vi "analyze data.vi"() -> ()   [LabVIEW 2014]
uses:
  <vilib>/Analysis/baseanly.llb/Mean (DBL).vi
  <vilib>/gmath/SpecialFunctions.llb/Factorial.vi
  <vilib>/Utility/file.llb/Read From Spreadsheet File (DBL).vi
  <vilib>/imath/engines/lvmath2/RunTimeEngine/Managers/WorkSpace/UID Generator.vi
  <vilib>/imath/engines/lvmath2/RunTimeEngine/RunTimeType/NIMS_RunTimeType_From StrictType (excl LVString).vi
  <instcachedir>/0/NIMS_RunTimeType_From StrictType (excl LVString)_15A5391EEA9C4AACB9955AC755B83D29.lvgen/NIMS_RunTimeType_From StrictType (excl LVString)_15A5391EEA9C4AACB9955AC755B83D29_000.vi
  <vilib>/imath/engines/lvmath2/RunTimeEngine/LocalVariableDefStatement/MC_LocalVariableDefStatement_Display.vi
  <vilib>/imath/engines/lvmath2/RunTimeEngine/BuiltInFunctions/max/1 input/NIMS_max(RV).vi
  <instcachedir>/0/NIMS_max(RV)_237633DB1D604D5BA7001287DF3C7957.lvgen/NIMS_max(RV)_237633DB1D604D5BA7001287DF3C7957_000.vi
  <vilib>/imath/engines/lvmath2/RunTimeEngine/Managers/SymbolTable/Clear UID.vi
  <vilib>/imath/engines/lvmath2/RunTimeEngine/NodeEndStatement/NIMS_NodeEndStatement_Output.vi
  <instcachedir>/0/NIMS_NodeEndStatement_Output_53EC0D466D134D7ABD903AC30B43404B.lvgen/NIMS_NodeEndStatement_Output_53EC0D466D134D7ABD903AC30B43404B_005.vi
  <instcachedir>/0/NIMS_NodeEndStatement_Output_53EC0D466D134D7ABD903AC30B43404B.lvgen/NIMS_NodeEndStatement_Output_53EC0D466D134D7ABD903AC30B43404B_004.vi
  <vilib>/imath/engines/lvmath2/RunTimeEngine/ErrorHandling/NIMS_Finalize Error.vi
  <vilib>/Analysis/NI_AALBase.lvlib
  <vilib>/gmath/NI_Gmath.lvlib
  <vilib>/imath/engines/lvmath2/RunTimeEngine/Managers/SymbolTable/NIMS_WorkSpace.lvlib
panel:
  out "?":dbl=44.2093023255814
  out "XY Graph 2":cluster{"X Values":dbl[], "yout":dbl[]}[](graph)=[{"X Values"=[3.05, 9.15, 15.25, 21.35, 27.45, 33.55, 39.65, 45.75, 51.85, 57.95], "yout"=[1.0, 0.0, 0.0, 0.0, 6.0, 30.0, 83.0, 101.0, 64.0, 16.0]}, {"X Values"=[1.0, 2.0, 3.0, 4.0, 5.0, 6.0, 7.0, 8.0, 9.0, 10.0, 11.0, 12.0, 13.0, 14.0, 15.0, 16.0, 17.0, 18.0, 19.0, 20.0, 21.0, 22.0, 23.0, 24.0, 25.0, 26.0, 27.0, 28.0, 29.0, 30.0, 31.0, 32.0, 33.0, 34.0, 35.0, 36.0, 37.0, 38.0, 39.0, 40.0, 41.0, 42.0, 43.0, 44.0, 45.0, 46.0, 47.0, 48.0, 49.0, 50.0, 51.0, 52.0, 53.0, 54.0, 55.0, 56.0, 57.0, 58.0, 59.0, 60.0], "yout"=[4.697137632968925e-15, 1.0382858884039449e-13, 1.530063158027829e-12, 1.691075618262153e-11, 1.4952254652634198e-10, 1.101714577312311e-09, 6.958004689271438e-09, 3.845106661135175e-08, 1.8887720317359093e-07, 8.350129377511543e-07, 3.3559399464375147e-06, 1.2363646973212627e-05, 4.204524668350126e-05, 0.00013277078728461114, 0.00039131359167138887, 0.0010812313048943463, 0.002811793037762178, 0.00690596713796628, 0.016068841529099022, 0.035519613659089816, 0.07477606374964532, 0.1502635276829554, 0.2888280749497454, 0.5320369868987074, 0.9408393600878537, 1.599763527305018, 2.619423312150594, 4.135817040197906, 6.304882272186222, 9.29114821660931, 13.250167111608626, 18.30564511567442, 24.52363027829251, 31.88742897334752, 40.27774251052069, 49.462524878875854, 59.10010043667066, 68.75721599149993, 77.94124484188515, 86.14320142117656, 92.88611792493289, 97.77215402840388, 100.52183061546553, 101.0, 99.22532299741601, 95.36265875535283, 89.70035343588606, 82.61645924497063, 74.53910252714248, 65.90643437399899, 57.13093102825904, 48.57151157635083, 40.51533282432774, 33.169529586152905, 26.66185020857364, 21.04824636482496, 16.32505766606783, 12.443438100719709, 9.323995202786033, 6.87012204670397]}]
  in  "Constant Data":path=path "U:/LabView/week8/constant.txt"
  out "Mean Lifetime":dbl=140.7967398239417
  out "XY Graph":cluster{"all rows":dbl[], "Array":dbl[]}[](graph)=[{"all rows"=[0.0, 1.0, 2.0, 3.0, 4.0, 5.0, 6.0, 7.0, 8.0, 9.0, 10.0, 11.0, 12.0, 13.0, 14.0, 15.0, 16.0, 17.0, 18.0, 19.0, 20.0, 21.0, 22.0, 23.0, 24.0, 25.0, 26.0, 27.0, 28.0, 29.0, 30.0, 31.0, 32.0, 33.0, 34.0, 35.0, 36.0, 37.0, 38.0, 39.0, 40.0, 41.0, 42.0, 43.0, 44.0, 45.0, 46.0, 47.0, 48.0, 49.0, 50.0, 51.0, 52.0, 53.0, 54.0, 55.0, 56.0, 57.0, 58.0, 59.0, 60.0, 61.0, 62.0, 63.0, 64.0, 65.0, 66.0, 67.0, 68.0, 69.0, 70.0, 71.0, 72.0, 73.0, 74.0, 75.0, 76.0, 77.0, 78.0, 79.0, 80.0, 81.0, 82.0, 83.0, 84.0, 85.0, 86.0, 87.0, 88.0, 89.0, 90.0, 91.0, 92.0, 93.0, 94.0, 95.0, 96.0, 97.0, 98.0, 99.0, 100.0, 101.0, 102.0, 103.0, 104.0, 105.0, 106.0, 107.0, 108.0, 109.0, 110.0, 111.0, 112.0, 113.0, 114.0, 115.0, 116.0, 117.0, 118.0, 119.0, 120.0, 121.0, 122.0, 123.0, 124.0, 125.0, 126.0, 127.0, 128.0, 129.0, 130.0, 131.0, 132.0, 133.0, 134.0, 135.0, 136.0, 137.0, 138.0, 139.0, 140.0, 141.0, 142.0, 143.0, 144.0, 145.0, 146.0, 147.0, 148.0, 149.0, 150.0, 151.0, 152.0, 153.0, 154.0, 155.0, 156.0, 157.0, 158.0, 159.0, 160.0, 161.0, 162.0, 163.0, 164.0, 165.0, 166.0, 167.0, 168.0, 169.0, 170.0, 171.0, 172.0, 173.0, 174.0, 175.0, 176.0, 177.0, 178.0, 179.0, 180.0, 181.0, 182.0, 183.0, 184.0, 185.0, 186.0, 187.0, 188.0, 189.0, 190.0, 191.0, 192.0, 193.0, 194.0, 195.0, 196.0, 197.0, 198.0, 199.0, 200.0, 201.0, 202.0, 203.0, 204.0, 205.0, 206.0, 207.0, 208.0, 209.0, 210.0, 211.0, 212.0, 213.0, 214.0, 215.0, 216.0, 217.0, 218.0, 219.0, 220.0, 221.0, 222.0, 223.0, 224.0, 225.0, 226.0, 227.0, 228.0, 229.0, 230.0, 231.0, 232.0, 233.0, 234.0, 235.0, 236.0, 237.0, 238.0, 239.0, 240.0, 241.0, 242.0, 243.0, 244.0, 245.0, 246.0, 247.0, 248.0, 249.0, 250.0, 251.0, 252.0, 253.0, 254.0, 255.0, 256.0, 257.0, 258.0, 259.0, 260.0, 261.0, 262.0, 263.0, 264.0, 265.0, 266.0, 267.0, 268.0, 269.0, 270.0, 271.0, 272.0, 273.0, 274.0, 275.0, 276.0, 277.0, 278.0, 279.0, 280.0, 281.0, 282.0, 283.0, 284.0, 285.0, 286.0, 287.0, 288.0, 289.0, 290.0, 291.0, 292.0, 293.0, 294.0, 295.0, 296.0, 297.0, 298.0, 299.0, 300.0], "Array"=[33.48144002446238, 33.24448268334883, 33.00920235437892, 32.775587168877394, 32.54362534216689, 32.313305172973415, 32.08461504283611, 31.857543415521167, 31.63207883643986, 31.408209932070736, 31.185925409385867, 30.96521405528119, 30.746064736010855, 30.528466396625596, 30.31240806041504, 30.097878828354023, 29.884867878552765, 29.673364465710968, 29.463357920575785, 29.25483764940359, 29.04779313342559, 28.842213928317204, 28.638089663671213, 28.435410042474604, 28.23416484058916, 28.034343906235687, 27.835937159481933, 27.638934591734085, 27.44332626523189, 27.249102312547365, 27.05625293608701, 26.86476840759759, 26.674639067675397, 26.48585532527895, 26.29840765724523, 26.112286607809242, 25.927482788127033, 25.74398687580208, 25.56178961441502, 25.380881813056703, 25.201254345864577, 25.02289815156232, 24.84580423300275, 24.669963656713954, 24.49536755244867, 24.3220071127368, 24.149873592441132, 23.97895830831619, 23.809252638570207, 23.640748022430206, 23.473435959710155, 23.30730801038216, 23.142355794150735, 22.97857099003003, 22.815945335924102, 22.654470628210138, 22.494138721324603, 22.334941527352356, 22.176871015618655, 22.019919212284037, 21.864078199942103, 21.709340117220098, 21.555697158382372, 21.403141572936605, 21.25166566524284, 21.10126179412526, 20.951922372486774, 20.80363986692624, 20.65640679735847, 20.510215736636894, 20.365059310178896, 20.220930195593805, 20.077821122313505, 19.935724871225712, 19.79463427430976, 19.654542214275047, 19.515441624201983, 19.377325487185505, 19.24018683598112, 19.104018752653428, 18.96881436822717, 18.834566862340697, 18.701269462901937, 18.56891544574677, 18.437498134299844, 18.30701089923774, 18.177447158154596, 18.048800375230044, 17.921064060899507, 17.794231771526835, 17.668297109079266, 17.54325372080466, 17.419095298911067, 17.295815580248494, 17.17340834599299, 17.051867421332922, 16.931186675157495, 16.81136001974748, 16.69238141046808, 16.57424484546407, 16.456944365356982, 16.340474052944508, 16.224828032902007, 16.110000471486128, 15.995985576240512, 15.882777595703615, 15.770370819118556, 15.658759576145052, 15.547938236573373, 15.437901210040335, 15.328642945747278, 15.220157932180078, 15.112440696831099, 15.005485805923149, 14.899287864135378, 14.793841514331083, 14.689141437287507, 14.585182351427475, 14.481959012552998, 14.37946621358071, 14.277698784279199, 14.176651591008207, 14.076319536459653, 13.976697559400504, 13.87778063441747, 13.779563771663474, 13.682042016605976, 13.585210449777005, 13.489064186525031, 13.39359837676853, 13.298808204751346, 13.204688888799744, 13.111235681081212, 13.01844386736495, 12.92630876678406, 12.834825731599434, 12.743990146965272, 12.653797430696324, 12.564243033036707, 12.47532243643042, 12.387031155293437, 12.299364735787451, 12.212318755595184, 12.125888823697311, 12.04007058015096, 11.95485969586977, 11.870251872405513, 11.786242841731255, 11.702828366026065, 11.620004237461234, 11.537766277988005, 11.456110339126832, 11.375032301758079, 11.294528075914267, 11.214593600573732, 11.135224843455775, 11.056417800817258, 10.978168497250623, 10.900472985483372, 10.82332734617894, 10.74672768773897, 10.670670146107023, 10.595150884573652, 10.52016609358285, 10.445711990539879, 10.371784819620473, 10.298380851581358, 10.225496383572143, 10.153127738948518, 10.081271267086803, 10.009923343199779, 9.939080368153839, 9.86873876828744, 9.798894995230812, 9.729545525726982, 9.660686861454026, 9.592315528848614, 9.524428078930763, 9.45702108712988, 9.390091153111992, 9.32363490060823, 9.257648977244495, 9.192130054372369, 9.127074826901191, 9.06248001313133, 8.998342354588646, 8.934658615860117, 8.871425584430623, 8.8086400705209, 8.746298906926627, 8.68439894885865, 8.62293707378436, 8.56191018127016, 8.501315192825087, 8.441149051745484, 8.381408722960836, 8.322091192880658, 8.263193469242466, 8.204712580960841, 8.146645577977546, 8.088989531112729, 8.031741531917133, 7.974898692525403, 7.918458145510397, 7.862417043738543, 7.806772560226216, 7.7515218879971295, 7.696662239940735, 7.642190848671633, 7.588104966389972, 7.534401864742834, 7.481078834686598, 7.428133186350296, 7.375562248899908, 7.323363370403647, 7.271533917698167, 7.220071276255748, 7.1689728500523975, 7.1182360614369, 7.067858351000779, 7.017837177449201, 6.968170017472771, 6.91885436562025, 6.869887734172157, 6.821267653015293, 6.772991669518124, 6.725057348407065, 6.677462271643629, 6.630204038302449, 6.583280264450172, 6.536688583025188, 6.49042664371824, 6.444492112853845, 6.398882673272591, 6.353596024214234, 6.308629881201645, 6.263981975925562, 6.219650056130174, 6.175631885499502, 6.131925243544592, 6.0885279254914915, 6.045437742170046, 6.002652519903456, 5.960170100398629, 5.917988340637309, 5.876105112767963, 5.834518303998449, 5.793225816489438, 5.7522255672485825, 5.711515488025444, 5.671093525207162, 5.630957639714854, 5.5911058069007655, 5.55153601644612, 5.512246272259727, 5.473234592377277, 5.43449900886137, 5.3960375677022325, 5.357848328719161, 5.319929365462641, 5.2822787651171685, 5.244894628404762, 5.207775069489151, 5.170918215880645, 5.134322208341677, 5.097985200793017, 5.061905360220642, 5.026080866583273, 4.990509912720562, 4.955190704261933, 4.920121459536061, 4.885300409480997, 4.850725797554934, 4.8163958796475885, 4.7823089239922245, 4.748463211078298, 4.7148570335647095, 4.681488696193685, 4.64835651570525, 4.615458820752325, 4.5827939518164165, 4.550360261123894, 4.518156112562872, 4.486179881600685, 4.454429955201926, 4.422904731747079, 4.391602620951737, 4.360522043786365, 4.3296614323966605, 4.2990192300244505, 4.268593890929167, 4.238383880309878, 4.208387674227853, 4.178603759529695, 4.1490306337710114, 4.11966680514062, 4.090510792385294, 4.061561124735046, 4.032816341828927, 4.004274993641368, 3.975935640409025]}, ...(2 in all)]
  in  "Decay Data":path=path "U:/LabView/week8/data.txt"
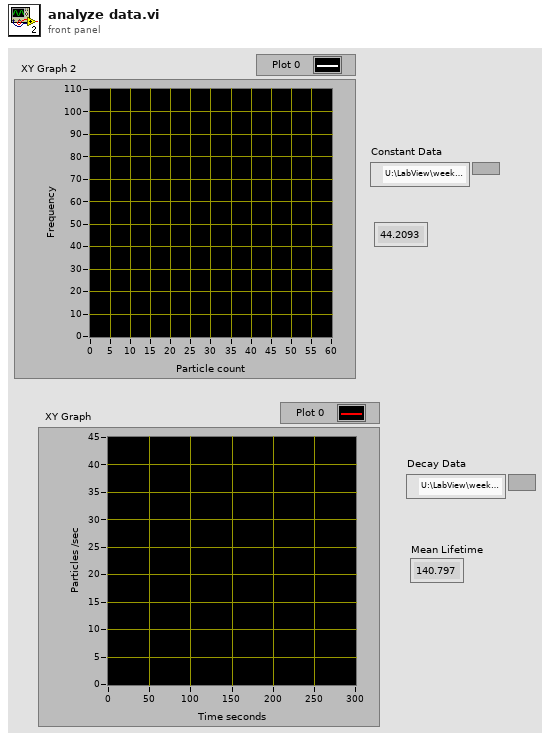
[diagram p1: front panel]
types:
  T1 = cluster{"X Values":dbl[], "Histogram: h(x)":i32[]}
  T2 = cluster{"Array[0]":dbl, "Array[1]":dbl, "Array[2]":dbl, "Array[3]":dbl, "Array[4]":dbl, "Array[5]":dbl, "Array[6]":dbl, "Array[7]":dbl, "Array[8]":dbl}
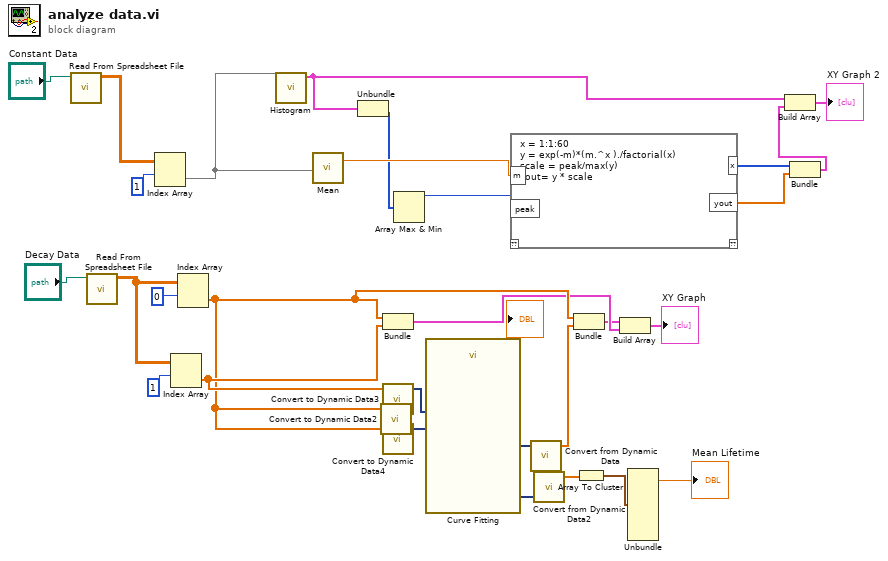
[diagram p0: block diagram]
diagram:
  n1 = call-poly <vilib>:"Read From Spreadsheet File.vi"("file path (dialog if empty)"="Constant Data") -> ("all rows"=w11:dbl[][])  [unwired: 6 in, 4 out]
  n2 = call-poly <vilib>:"Read From Spreadsheet File.vi"("file path (dialog if empty)"="Decay Data") -> ("all rows"=w27:dbl[][])  [unwired: 6 in, 4 out]
  n3 = Index Array(array=w11, index (row)=1) -> (element=w5:dbl[])  [unwired: 1 in]
  n4 = Index Array(array=w27, index (row)=1) -> (element=w21:dbl[])  [unwired: 1 in]
  n5 = Index Array(array=w27, index (row)=0) -> (element=w19:dbl[])  [unwired: 1 in]
  n6 = call <vilib>:"Histogram.vi"("X"=w5) -> ("Histogram Graph"=w2:T1)  [unwired: 7 in, 3 out]
  n7 = call-poly <vilib>:"Mean.vi"("X"=w5) -> ("mean"=w6:dbl)  [unwired: 1 out]
  n8 = Unbundle(w2) -> ("Histogram: h(x)"=w3:i32[])  [unwired: 1 out]
  n9 = call "Convert to Dynamic Data2"("Array"=w19) -> ()  [unwired: 3 in, 1 out]
  n10 = Bundle("all rows"=w19, "all rows"=w21) -> (w18:cluster{"all rows":dbl[], "all rows":dbl[]})  [unwired: 1 in]
  n11 = call "Convert to Dynamic Data3"("Array"=w21) -> ("Dynamic Data Type"=w25:dynamicdata)  [unwired: 3 in]
  n12 = call "Convert to Dynamic Data4"("Array"=w19) -> ("Dynamic Data Type"=w24:dynamicdata)  [unwired: 3 in]
  n13 = Array Max & Min(array=w3) -> (max value=w4:i32)  [unwired: 3 out]
  n14 = call "Curve Fitting"("Locations"=w24, "Signals"=w25) -> ("best fit"=w23:dynamicdata, "non-linear coefficients"=w16:dynamicdata)  [unwired: 5 in, 3 out]
  n15 = mathscript code="x = 1:1:60\ny = exp(-m)*(m.^x )./factorial(x) \nscale = peak/max(y)\nyout= y * scale"("m"=w6, "peak"=w4) -> ("x"=w9:i32[], "yout"=w7:dbl[])  [unwired: 1 in, 1 out]
  n16 = call "Convert from Dynamic Data"("Dynamic Data Type"=w23) -> ("Array"=w22:dbl[])  [unwired: 3 in]
  n17 = call "Convert from Dynamic Data2"("Dynamic Data Type"=w16) -> ("Array"=w15:dbl[])  [unwired: 3 in]
  n18 = Bundle("all rows"=w19, "Array"=w22) -> (w17:cluster{"all rows":dbl[], "Array":dbl[]})  [unwired: 1 in]
  n19 = Array To Cluster(array=w15) -> (cluster=w14:T2)
  n20 = Build Array(w17, w18) -> (→"XY Graph":cluster{"all rows":dbl[], "all rows":dbl[]}[])
  n21 = Unbundle(w14) -> ("Array[1]"=→"Mean Lifetime":dbl)  [unwired: 8 out]
  n22 = Bundle("x"=w9, "yout"=w7) -> (w1:cluster{"x":i32[], "yout":dbl[]})  [unwired: 1 in]
  n23 = Build Array(w2, w1) -> (→"XY Graph 2":cluster{"X Values":dbl[], "yout":dbl[]}[])
